vi "Yield Error.vi"(0 "WAMP Client in":refnum<class "WAMP Client.lvclass">, 5 "Invocation Request ID":u32, 7 "Error URI":string, 9 "ArgumentsKw":string, 11 "error in (no error)":errorcluster, 12 "Arguments Payload":string[](array[string]), 13 "Details":string) -> (4 "WAMP Client out":refnum<class "WAMP Client.lvclass">, 15 "error out":errorcluster)   [LabVIEW 2020, in "wamplv.lvlib" / "WAMP Client.lvclass"]
uses:
  <vilib>/samangh/wamplv/WAMP Client/WAMP Client.lvclass
  <vilib>/samangh/wamplv/WAMP Client/TypeDef/WAMP Error Payload.ctl
  <vilib>/samangh/wamplv/WAMP Message Codes.ctl
  <vilib>/samangh/wamplv/WAMP Client/TypeDef/Error Request.ctl
  <vilib>/samangh/wamplv/WAMP Client/TypeDef/Internal Message Type.ctl
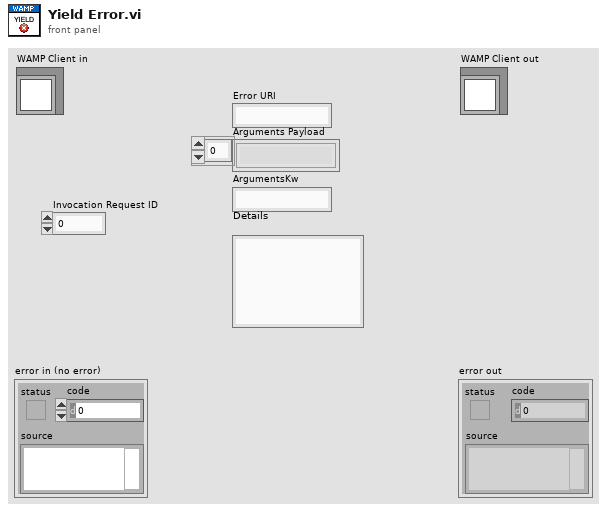
[diagram p1: front panel]
types:
  T1 = typedef "wamplv.lvlib/WAMP Client.lvclass/WAMP Error Payload.ctl" = cluster{"Details":string, "ArgumentKw Payload":string, "Error?":bool, "Error URI":string, "Arguments Payload":string[]}
  T2 = typedef "wamplv.lvlib/WAMP Client.lvclass/Error Request.ctl" = cluster{"WAMP Error":T1, "Message Type":T3, "Request ID":u64}
  T3 = typedef "wamplv.lvlib/WAMP Client.lvclass/WAMP Message Codes.ctl" = u16
  T4 = typedef "wamplv.lvlib/WAMP Client.lvclass/Internal Message Type.ctl" = enum16{"Subscribe", "Handle Subscribed", "Handle Event", "Unsubscribe", "Handle Unsubscribed", "Publish", "Handled Published", "Goodbye", "Handle Goodbye", "Call", "Handle Result", "Register", "Handle Registered", "Unregister", "Handle Unregistered", "Handle Invocation", "Yield", "Error"}
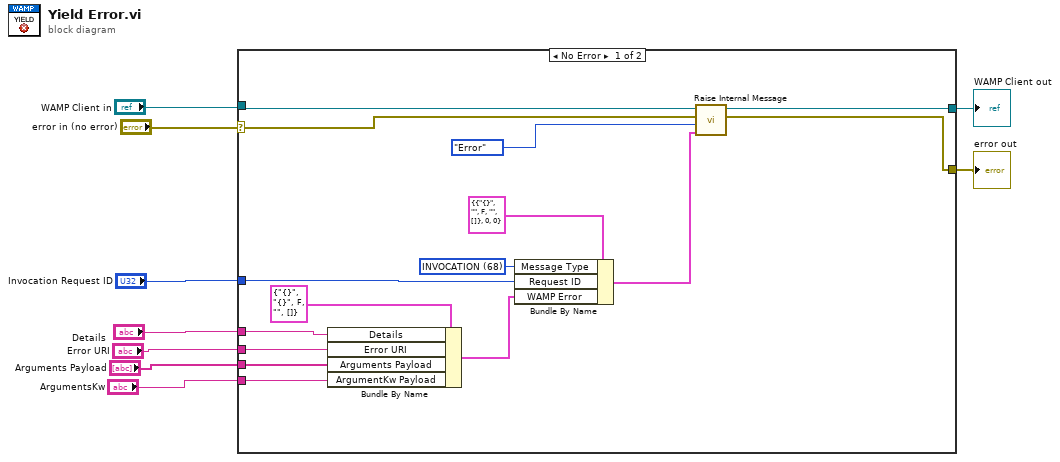
[diagram p0: block diagram]
diagram:
  n1 = case shown="No Error" "error in (no error)" {
    selector: "error in (no error)" -> [w20 w26]
    tunnel: [w21 w26] -> w8
    tunnel: [w23 w25] -> w6
    tunnel: "WAMP Client in" -> [w24 w25]
    tunnel: "ArgumentsKw" -> [w14 _]
    tunnel: "Invocation Request ID" -> [w17 _]
    tunnel: "Details" -> [w15 _]
    tunnel: "Error URI" -> [w13 _]
    tunnel: "Arguments Payload" -> [w12 _]
    frame No Error {
      w18 = T3 68 items=["HELLO"=1, "WELCOME"=2, "ABORT"=3, "GOODBYE"=6, "ERROR"=8, "PUBLISH"=16, "PUBLISHED"=17, "SUBSCRIBE"=32, "SUBSCRIBED"=33, "UNSUBSCRIBE"=34, "UNSUBSCRIBED"=35, "EVENT"=36, "CALL"=48, "RESULT"=59, "REGISTER"=64, "REGISTERED"=65, "UNREGISTER"=66, "UNREGISTERED"=67, "INVOCATION"=68, "YIELD"=70] ("Message Type")
      n2 = Bundle By Name(cluster=T1 {"Details"="{}", "ArgumentKw Payload"="{}", "Error?"=FALSE, "Error URI"="", "Arguments Payload"=[]} ("WAMP Error"), "Details"=w15, "Error URI"=w13, "Arguments Payload"=w12, "ArgumentKw Payload"=w14) -> (w11:T1)
      n3 = Bundle By Name(cluster=T2 {"WAMP Error"={"Details"="{}", "ArgumentKw Payload"="", "Error?"=FALSE, "Error URI"="", "Arguments Payload"=[]}, "Message Type"=0, "Request ID"=0} ("Error Request"), "Message Type"=w18, "Request ID"=w17, "WAMP Error"=w11) -> (w10:T2)
      n4 = call-dynamic "Raise Internal Message.vi"("Variant"=w10, "Internal Message Type"=Internal_Message_Type."Error", "error in (no error)"=w20, "WAMP Client in"=w24) -> ("error out"=w21:errorcluster, "WAMP Client out"=w23:refnum<class "WAMP Client.lvclass">)  [unwired: 6 in]
    }
    frame Error {
    }
  }
  "error out" <- w8
  "WAMP Client out" <- w6
